vi "setFilter.vi"(8 "error in (no error)":errorcluster, 11 "Electrometer in":refnum<class "Electrometer.lvclass">) -> (0 "error out":errorcluster, 3 "Electrometer out":refnum<class "Electrometer.lvclass">)   [LabVIEW 2016, in "Electrometer.lvclass"]
uses:
  Electrometer.lvclass
  filterType.ctl
  ElectrometerConfiguration/ElectrometerInternalConfiguration.lvclass
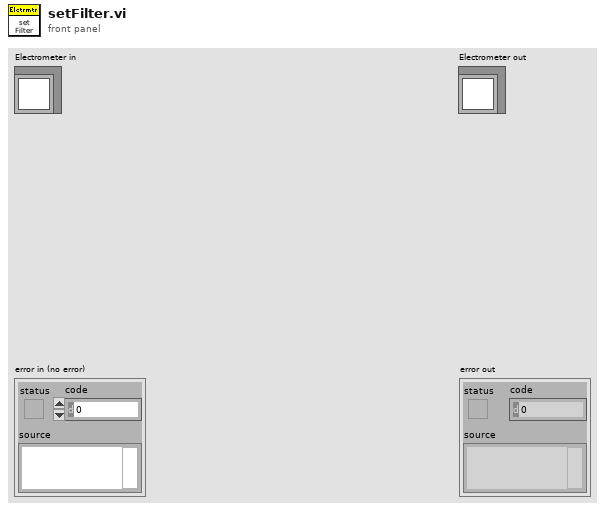
[diagram p1: front panel]
types:
  T1 = typedef "Electrometer.lvclass/filterType.ctl" = enum16{"Median", "Average"}
  T2 = typedef "Electrometer.lvclass/MED Filter Type.ctl" = enum16{"Active", "None"}
  T3 = typedef "Electrometer.lvclass/Modes.ctl" = enum16{"Current", "Charge", "Voltage", "Resistance"}
  T4 = typedef "Electrometer.lvclass/AVG Filter type.ctl" = enum16{"None", "Scalar", "Advanced"}
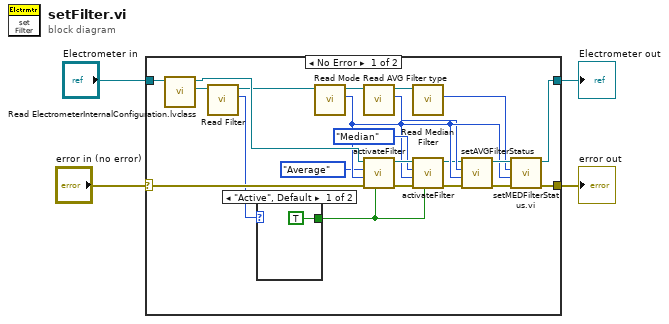
[diagram p0: block diagram]
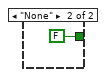
[diagram p2: hidden frame]
diagram:
  n1 = case shown="No Error" "error in (no error)" {
    selector: "error in (no error)" -> [w22 w30]
    tunnel: [w23 w30] -> w3
    tunnel: [w25 w29] -> w1
    tunnel: "Electrometer in" -> [w26 w29]
    frame No Error {
      n2 = call-dynamic "Read ElectrometerInternalConfiguration.lvclass.vi"("Electrometer in"=w26) -> ("ElectrometerInternalConfiguration.lvclass"=w6:refnum<class "ElectrometerInternalConfiguration.lvclass">, "Electrometer out"=w21:refnum<class "Electrometer.lvclass">)  [unwired: 8 in, 1 out]
      n3 = call-dynamic "Read Filter.vi"("ElectrometerInternalConfiguration in"=w6) -> ("Filter"=w19:T2, "ElectrometerInternalConfiguration out"=w5:refnum<class "ElectrometerInternalConfiguration.lvclass">)  [unwired: 8 in, 1 out]
      n4 = case shown="\"Active\", Default" w19 {
        tunnel: [TRUE FALSE] -> w16
        frame "Active", Default {
        }
        frame "None" {
        }
      }
      n5 = call-dynamic "Read Mode.vi"("ElectrometerInternalConfiguration in"=w5) -> ("Measurement Function (0: Current)"=w14:T3, "ElectrometerInternalConfiguration out"=w8:refnum<class "ElectrometerInternalConfiguration.lvclass">)  [unwired: 8 in, 1 out]
      n6 = call-dynamic "Read AVG Filter type.vi"("ElectrometerInternalConfiguration in"=w8) -> ("AVG Filter type"=w11:T4, "ElectrometerInternalConfiguration out"=w7:refnum<class "ElectrometerInternalConfiguration.lvclass">)  [unwired: 8 in, 1 out]
      n7 = call-dynamic "activateFilter.vi"("Activate"=w16, "error in (no error)"=w22, "Measurement Function"=w14, "Filter Type"=filterType."Average", "Electrometer in"=w21) -> ("error out"=w18:errorcluster, "Electrometer out"=w17:refnum<class "Electrometer.lvclass">)  [unwired: 5 in]
      n8 = call-dynamic "Read Median Filter.vi"("ElectrometerInternalConfiguration in"=w7) -> ("Filter"=w12:T2)  [unwired: 8 in, 2 out]
      n9 = call-dynamic "activateFilter.vi"("Activate"=w16, "error in (no error)"=w18, "Measurement Function"=w14, "Filter Type"=filterType."Median", "Electrometer in"=w17) -> ("error out"=w9:errorcluster, "Electrometer out"=w10:refnum<class "Electrometer.lvclass">)  [unwired: 5 in]
      n10 = call-dynamic "setAVGFilterStatus.vi"("error in (no error)"=w9, "Measurement Function (0: Current)"=w14, "AVG Filter type"=w11, "Electrometer in"=w10) -> ("error out"=w24:errorcluster, "Electrometer out"=w20:refnum<class "Electrometer.lvclass">)  [unwired: 6 in]
      n11 = call-dynamic "setMEDFilterStatus.vi.vi"("error in (no error)"=w24, "Measurement Function (0: Current)"=w14, "MED Filter Active"=w12, "Electrometer in"=w20) -> ("error out"=w23:errorcluster, "Electrometer out"=w25:refnum<class "Electrometer.lvclass">)  [unwired: 6 in]
    }
    frame Error {
    }
  }
  "error out" <- w3
  "Electrometer out" <- w1
